vi "FindMaxRate.vi"(8 "error in (no error)":errorcluster, 10 "Current (A)":dbl format="%#_13g", 11 "PS Driver in":refnum<class "PS Driver.lvclass">) -> (0 "error out":errorcluster, 2 "Max rate (A/sec)":dbl, 3 "PS Driver out":refnum<class "PS Driver.lvclass">)   [LabVIEW 2025, in "PS Driver.lvlib" / "PS Driver.lvclass"]
doc: "Author: Scott Hannahs <sth@magnet.fsu.edu>\n\nThis software is licensed for use under the “MIT License\"\nCopyright (c) 2025 Scott Hannahs, sth@sth@magnet.sthnet.net\n\nPermission is hereby granted, free of charge, to any person obtaining a copy of this software and associated documentation files (the \"Software\"), to deal in the Software without restriction, including without limitation the rights to use, copy, modify, merge, publish, distribute, sublicense, and/or sell copies of the Software, and to permit persons to whom the Software is furnished to do so, subject to the following conditions: The above copyright notice and this permission notice shall be included in all copies or substantial portions of the Software.\n\nTHE SOFTWARE IS PROVIDED \"AS IS\", WITHOUT WARRANTY OF ANY KIND, EXPRESS OR IMPLIED, INCLUDING BUT NOT LIMITED TO THE WARRANTIES OF MERCHANTABILITY, FITNESS FOR A PARTICULAR PURPOSE AND NONINFRINGEMENT. IN NO EVENT SHALL THE AUTHORS OR COPYRIGHT HOLDERS BE LIABLE FOR ANY CLAIM, DAMAGES OR OTHER LIABILITY, WHETHER IN AN ACTION OF CONTRACT, TORT OR OTHERWISE, ARISING FROM, OUT OF OR IN CONNECTION WITH THE SOFTWARE OR THE USE OR OTHER DEALINGS IN THE SOFTWARE."
uses:
  PS Driver.lvclass
  PS Driver.lvclass/PS Driver.ctl
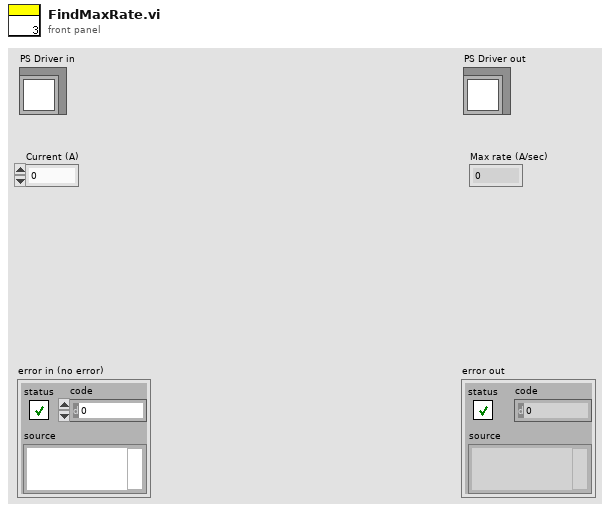
[diagram p1: front panel]
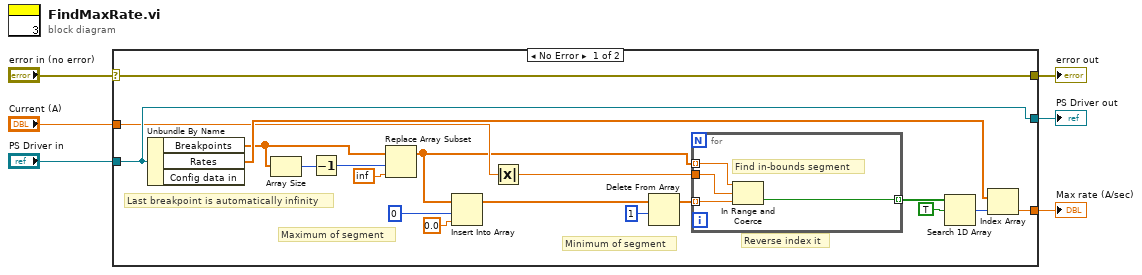
[diagram p0: block diagram]
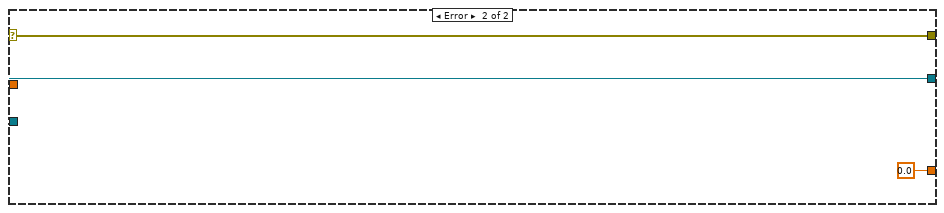
[diagram p2: hidden frame]
diagram:
  n1 = case shown="No Error" "error in (no error)" {
    selector: "error in (no error)" -> [w17 w32]
    tunnel: [w17 w32] -> w5
    tunnel: [w25 w31] -> w3
    tunnel: "PS Driver in" -> [w25 w31]
    tunnel: "Current (A)" -> [w15 _]
    tunnel: [w16 0.0] -> w1
    frame No Error {
      # "Last breakpoint is automatically infinity"
      # "Reverse index it"
      # "Maximum of segment"
      # "Minimum of segment"
      n2 = Unbundle By Name(w25) -> ("Breakpoints"=w12:dbl[], "Rates"=w18:dbl[])  [unwired: 1 out]
      n3 = Array Size(array=w12) -> (size(s)=w11:i32)
      n4 = Decrement(x=w11) -> (x-1=w10:i32)
      n5 = Replace Array Subset(array=w12, new element=inf, index=w10) -> (w9:dbl[])
      n6 = Insert Into Array(array=w9, index=0, new element=0.0 ("new element/subarray")) -> (w8:dbl[])
      n7 = Absolute Value(x=w15) -> (abs(x)=w14:dbl)
      n8 = Delete From Array(array=w8, length=1) -> (array with subset deleted=w7:dbl[])  [unwired: 1 in, 1 out]
      n9 = for {
        tunnel: w14 -> [w29]
        tunnel: w9 -> [w28] mode=indexing
        tunnel: w7 -> [w27] mode=indexing
        tunnel: [w26] -> w21 mode=indexing
        # "Find in-bounds segment"
        n10 = In Range and Coerce(upper limit=w28, x=w29, lower limit=w27) -> (In Range?=w26:bool)  [unwired: 1 out]
      }
      n11 = Search 1D Array(1D array=w21, element=TRUE) -> (index of element=w19:i32)  [unwired: 1 in]
      n12 = Index Array(array=w18, index=w19) -> (element=w16:dbl)
    }
    frame Error {
    }
  }
  "error out" <- w5
  "PS Driver out" <- w3
  "Max rate (A/sec)" <- w1
